vi "Get Master Resource and Channel.vi"(8 "error in (no error)":errorcluster, 9 "Channel modes":enum32{"Master", "Slave", "Slave - Inverted"}[](array[ring]), 10 "Channel names":string[](array[string]), 11 "Resource names":string[](array[string])) -> (0 "error out":errorcluster, 2 "Master channel name":string, 3 "Master resource name":string)   [LabVIEW 2021]
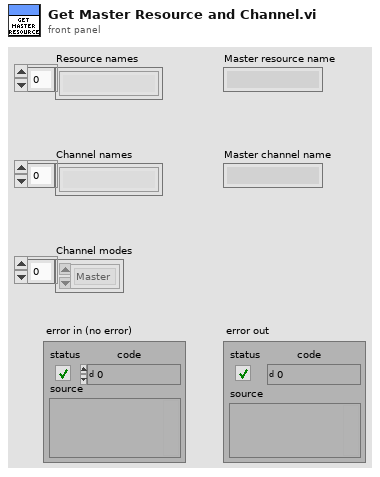
[diagram p1: front panel]
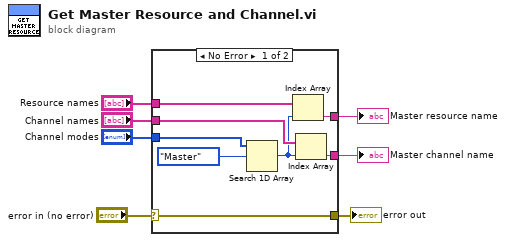
[diagram p0: block diagram]
diagram:
  n1 = case shown="No Error" "error in (no error)" {
    selector: "error in (no error)" -> [w8 w16]
    tunnel: "Resource names" -> [w15 _]
    tunnel: "Channel names" -> [w14 _]
    tunnel: "Channel modes" -> [w13 _]
    tunnel: [w12 _] -> w4
    tunnel: [w11 _] -> w3
    tunnel: [w8 w16] -> w1
    frame No Error {
      n2 = Search 1D Array(1D array=w13, element=enum32{"Master", "Slave", "Slave - Inverted"}."Master") -> (index of element=w10:i32)  [unwired: 1 in]
      n3 = Index Array(array=w15, index=w10) -> (element=w11:string)
      n4 = Index Array(array=w14, index=w10) -> (element=w12:string)
    }
    frame Error {
    }
  }
  "Master channel name" <- w4
  "Master resource name" <- w3
  "error out" <- w1
